vi "average-loop-time.vi"(9 "no-samples":i32=10, 11 "average-loop-time-cluster-in":T1) -> (0 "Loop Timing  Ave (mS)":dbl format="%.2f", 1 "Loop Timing (mS)":u32, 3 "average-loop-time-cluster-out":T1, 5 "array size":i32, 7 "sum of elements":u32)   [LabVIEW 2024]
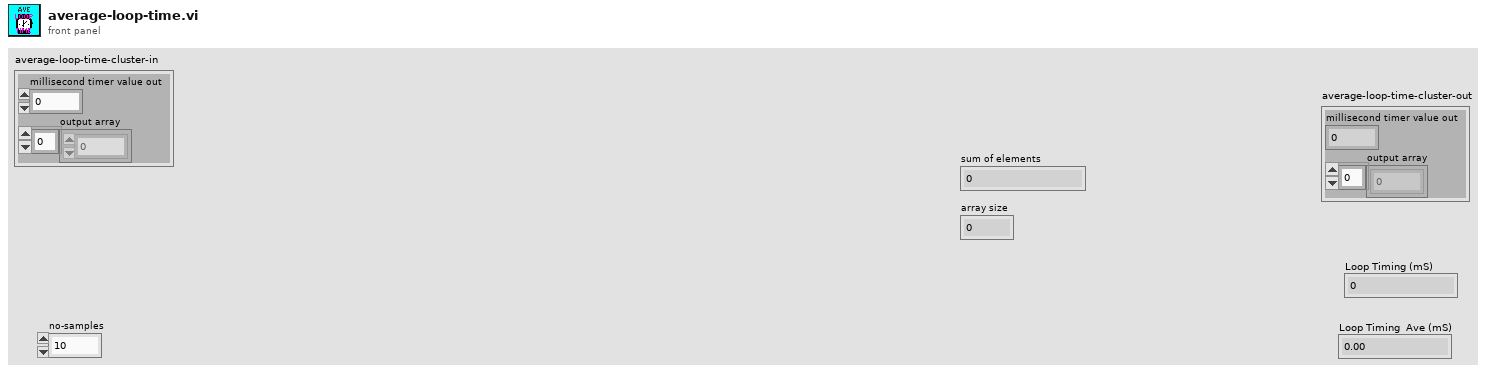
[diagram p1: front panel]
types:
  T1 = cluster{"millisecond timer value out":u32, "output array":u32[]}
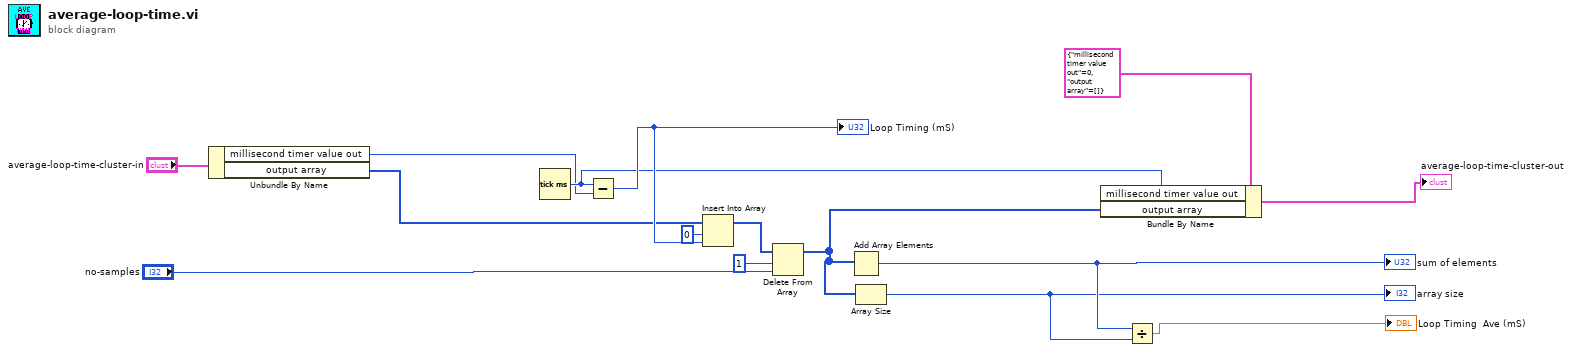
[diagram p0: block diagram]
diagram:
  n1 = Unbundle By Name("average-loop-time-cluster-in") -> ("millisecond timer value out"=w5:u32, "output array"=w2:u32[])
  n2 = Tick Count (ms)() -> (millisecond timer value=w7:u32)
  n3 = Subtract(x=w7, y=w5) -> (x-y=w15:u32)
  "Loop Timing (mS)" <- w15
  n4 = Insert Into Array(array=w2, index=0, new element=w15) -> (w8:u32[])
  n5 = Delete From Array(array=w8, length=1, index="no-samples") -> (array with subset deleted=w1:u32[])  [unwired: 1 out]
  n6 = Add Array Elements(numeric array=w1) -> (sum=w11:u32)
  "sum of elements" <- w11
  n7 = Array Size(array=w1) -> (size(s)=w10:i32)
  "array size" <- w10
  n8 = Bundle By Name(cluster=T1 {"millisecond timer value out"=0, "output array"=[]} ("average-loop-time-cluster-out"), "millisecond timer value out"=w7, "output array"=w1) -> (→"average-loop-time-cluster-out":T1)
  n9 = Divide(x=w11, y=w10) -> (x/y=→"Loop Timing  Ave (mS)":dbl)
